vi "RSLDiff.vi"() -> ()   [LabVIEW 2019]
panel:
  out "error out":errorcluster
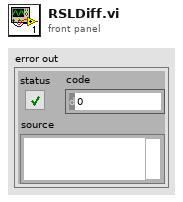
[diagram p1: front panel]
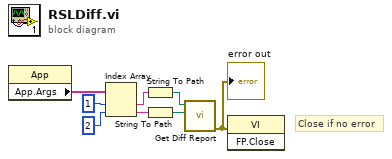
[diagram p0: block diagram]
diagram:
  # "Close if no error"
  n1 = property class="App"() -> ("App.Args"=w4:string[])  [unwired: 2 in, 2 out]
  n2 = Index Array(array=w4, index #1=1 ("index"), index #2=2 ("index")) -> (element #1=w8:string, element #2=w7:string)
  n3 = String To Path(string=w8) -> (path=w2:path)
  n4 = String To Path(string=w7) -> (path=w3:path)
  n5 = call "Get Diff Report.vi"("RSL Path"=w3, "Ref RSL Path"=w2) -> ("error out"=w1:errorcluster)  [unwired: 9 in]
  "error out" <- w1
  n6 = invoke class="VI" method="FP.Close"(error in=w1) -> ()  [unwired: 2 in, 3 out]
